vi "sel_obj.vi"(3 "error in":errorcluster, 4 "Object":string="Безымянный" caption="Объект", 5 "DevNo":u32, 6 "conn ref in":T1) -> (0 "error out":errorcluster, 1 "conn ref out":T1, 2 "Obj Id":i32)   [LabVIEW 2010]
uses:
  <vilib>/Addons/database/Connection.llb/Conn ObjectReference.ctl
  <vilib>/addons/database/_DB Variant To Data/Database Variant To Data.xnode
  <vilib>/addons/database/NI_Database_API.lvlib
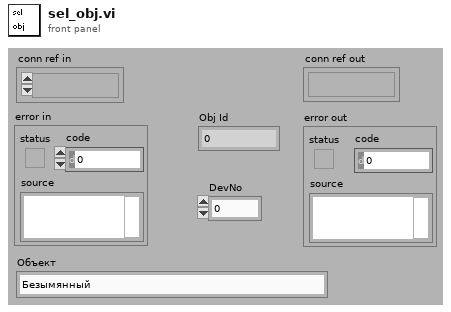
[diagram p1: front panel]
types:
  T1 = typedef "NI_Database_API.lvlib/Conn ObjectReference.ctl" = refnum<k1>
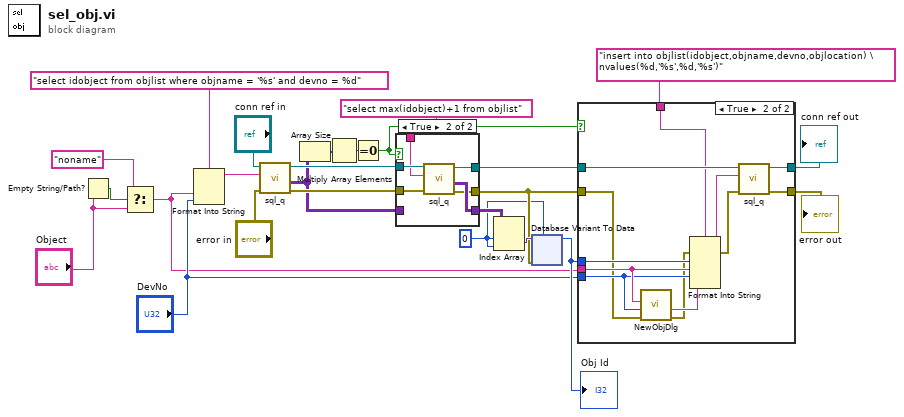
[diagram p0: block diagram]
diagram:
  w5 = 0 ("index (row)")
  n1 = Empty String/Path?(string/path="Object") -> (empty?=w4:bool)
  n2 = Select(t="noname", s=w4, f="Object") -> (s? t:f=w2:string)
  n3 = Format Into String(format string="select idobject from objlist where objname = '%s' and devno = %d" ("table"), w2, "DevNo") -> (resulting string=w17:string)  [unwired: 2 in, 1 out]
  n4 = call "sql_q.vi"("error in"="error in", "SQL query"=w17, "connect ref"="conn ref in") -> ("error out"=w20:errorcluster, "recordset data"=w11:variant[][], "conn ref out"=w21:T1)  [unwired: 1 in, 1 out]
  n5 = Array Size(array=w11) -> (size(s)=w25:i32[])
  n6 = Multiply Array Elements(1:w25) -> (0:w24:i32)
  n7 = Equal To 0?(x=w24) -> (x = 0?=w10:bool)
  n8 = case shown="True" w10 {
    tunnel: w21 -> [w28 w34]
    tunnel: w20 -> [w27 w33]
    tunnel: "select max(idobject)+1 from objlist" ("table") -> [_ w32]
    tunnel: [w26 w31] -> w14
    tunnel: [w28 w30] -> w12
    tunnel: [w27 w29] -> w7
    tunnel: w11 -> [w26 _]
    frame False {
    }
    frame True {
      n9 = call "sql_q.vi"("error in"=w33, "SQL query"=w32, "connect ref"=w34) -> ("error out"=w29:errorcluster, "recordset data"=w31:variant[][], "conn ref out"=w30:T1)  [unwired: 1 in, 1 out]
    }
  }
  n10 = Index Array(array=w14, index (row)=w5, index (col)=w5) -> (element=w13:variant)
  n11 = xnode "Database Variant To Data"("database variant"=w13, "error in"=w7, "type"=w5) -> ("data"=w8:i32)  [unwired: 1 out]
  "Obj Id" <- w8
  n12 = case shown="True" w10 {
    tunnel: [w36 w48] -> w16
    tunnel: [w35 w47] -> w15
    tunnel: w12 -> [w36 w46]
    tunnel: w7 -> [w35 w39]
    tunnel: "insert into objlist(idobject,objname,devno,objlocation) \nvalues(%d,'%s',%d,'%s')" ("table") -> [_ w44]
    tunnel: w2 -> [_ w41]
    tunnel: "DevNo" -> [_ w40]
    tunnel: w8 -> [_ w43]
    frame False {
    }
    frame True {
      n13 = call "NewObjDlg.vi"("error in (no error)"=w39, "DevNo"=w40, "ObjName"=w41) -> ("error out"=w38:errorcluster, "ObjLocation"=w42:string)  [unwired: 2 in, 1 out]
      n14 = Format Into String(format string=w44, error in=w38, w43, w41, w40, w42) -> (resulting string=w45:string, error out=w37:errorcluster)  [unwired: 1 in]
      n15 = call "sql_q.vi"("error in"=w37, "SQL query"=w45, "connect ref"=w46) -> ("error out"=w47:errorcluster, "conn ref out"=w48:T1)  [unwired: 1 in, 2 out]
    }
  }
  "error out" <- w15
  "conn ref out" <- w16
